vi "Animated 2.vi"() -> ()   [LabVIEW 2014, in "Arduino TFT.lvlib"]
uses:
  <vilib>/Aledyne-TSXperts/Arduino Compatible Compiler for LabVIEW/addons/Arduino TFT/Arduino TFT.lvlib
  <vilib>/Aledyne-TSXperts/Arduino Compatible Compiler for LabVIEW/Arduino Compatible Compiler for LabVIEW.lvlib
panel:
  in  "Error In":errorcluster
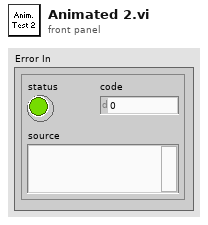
[diagram p1: front panel]
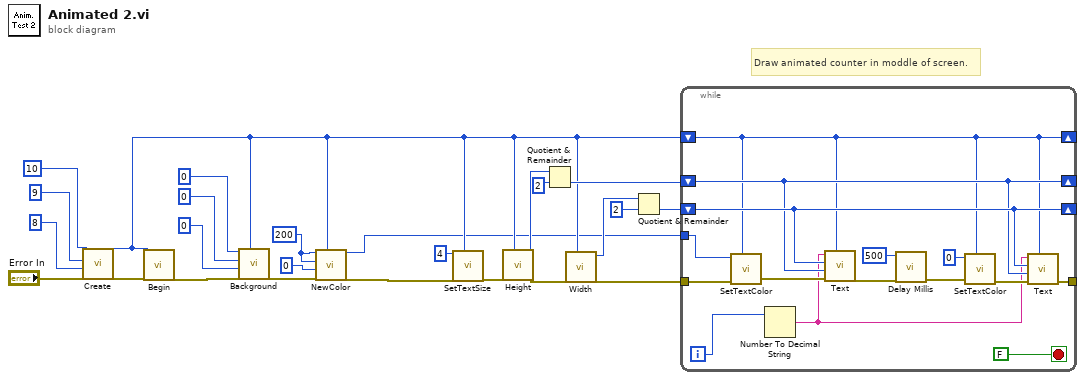
[diagram p0: block diagram]
diagram:
  w7 = u8 200 ("blue")
  # "Draw animated counter in moddle of screen."
  n1 = call <vilib>:"Create.vi"("Error In"="Error In", "rst"=u8 8 ("cs"), "rs"=u8 9 ("cs"), "cs"=u8 10) -> ("Error Out"=w21:errorcluster, "Instance"=w3:u32)  [unwired: 4 in]
  n2 = call <vilib>:"Begin.vi"("Error In"=w21, "Instance"=w3) -> ("Error Out"=w20:errorcluster)  [unwired: 8 in]
  n3 = call <vilib>:"Background.vi"("Instance"=w3, "Error In"=w20, "blue"=u8 0 ("red"), "green"=u8 0 ("red"), "red"=u8 0) -> ("Error Out"=w9:errorcluster)  [unwired: 6 in]
  n4 = call <vilib>:"NewColor.vi"("Instance"=w3, "Error In"=w9, "blue"=u8 0, "green"=w7, "red"=w7) -> ("Error Out"=w2:errorcluster, "color"=w1:u16)  [unwired: 5 in]
  n5 = call <vilib>:"SetTextSize.vi"("Instance"=w3, "Error In"=w2, "size"=u8 4) -> ("Error Out"=w14:errorcluster)  [unwired: 8 in]
  n6 = call <vilib>:"Height.vi"("Instance"=w3, "Error In"=w14) -> ("Error Out"=w15:errorcluster, "height"=w13:i16)  [unwired: 8 in]
  n7 = Quotient & Remainder(x=w13, y=i16 2) -> (floor(x/y)=w5:i16)  [unwired: 1 out]
  n8 = call <vilib>:"Width.vi"("Instance"=w3, "Error In"=w15) -> ("Error Out"=w6:errorcluster, "height"=w11:i16)  [unwired: 8 in]
  n9 = Quotient & Remainder(x=w11, y=i16 2) -> (floor(x/y)=w4:i16)  [unwired: 1 out]
  n10 = while {
    tunnel: w6 -> [w33]
    shift-right: [w28] -> _
    shift-left: w5 -> [w28]
    shift-right: [w29] -> _
    shift-left: w4 -> [w29]
    shift-right: [w26] -> _
    shift-left: w3 -> [w26]
    tunnel: w1 -> [w36]
    tunnel: [w30] -> _
    i -> [w40]
    stop <- FALSE stop-if-true
    n11 = call <vilib>:"SetTextColor.vi"("Instance"=w26, "Error In"=w33, "color"=w36) -> ("Error Out"=w34:errorcluster)  [unwired: 8 in]
    n12 = Number To Decimal String(number=w40) -> (decimal integer string=w27:string)  [unwired: 1 in]
    n13 = call <vilib>:"Text.vi"("Instance"=w26, "Error In"=w34, "y"=w28, "x"=w29, "text"=w27) -> ("Error Out"=w38:errorcluster)  [unwired: 6 in]
    n14 = call <vilib>:"Delay Millis.vi"("error in (no error)"=w38, "delay"=u32 500) -> ("error out"=w35:errorcluster)  [unwired: 9 in]
    n15 = call <vilib>:"SetTextColor.vi"("Instance"=w26, "Error In"=w35, "color"=u16 0) -> ("Error Out"=w31:errorcluster)  [unwired: 8 in]
    n16 = call <vilib>:"Text.vi"("Instance"=w26, "Error In"=w31, "y"=w28, "x"=w29, "text"=w27) -> ("Error Out"=w30:errorcluster)  [unwired: 6 in]
  }
